vi "Set Security Level CORE.vi"(8 "error in (no error)":errorcluster, 9 "Set or Clear":T1, 10 "New Level":T2, 11 "Security System in":refnum<class "Security System.lvclass">) -> (0 "error out":errorcluster, 2 "Last Action Performed":string, 3 "Security System out":refnum<class "Security System.lvclass">)   [LabVIEW 2014, in "Security System.lvclass"]
uses:
  Security System.lvclass
  Security Level.ctl
  Set or Clear.ctl
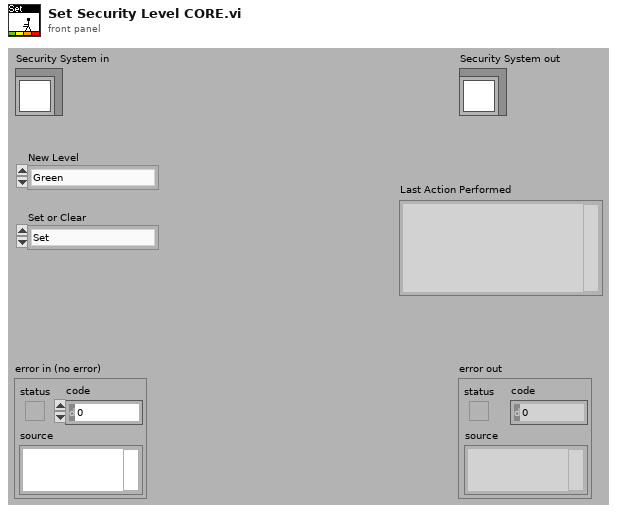
[diagram p1: front panel]
types:
  T1 = typedef "Security System.lvclass/Set or Clear.ctl" = enum16{"Set", "Clear"}
  T2 = typedef "Security System.lvclass/Security Level.ctl" = enum16{"Green", "Yellow", "Orange", "Red"}
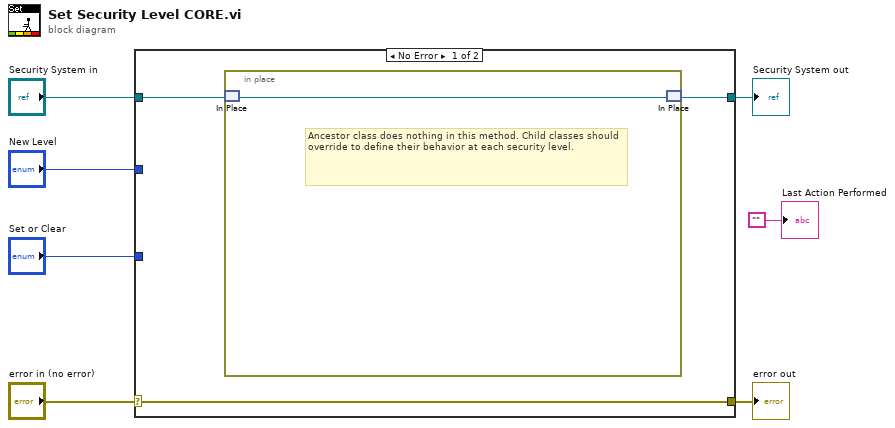
[diagram p0: block diagram]
diagram:
  n1 = case shown="No Error" "error in (no error)" {
    selector: "error in (no error)" -> [w10 w13]
    tunnel: [w10 w13] -> w6
    tunnel: [w8 w12] -> w4
    tunnel: "Security System in" -> [w9 w12]
    tunnel: "New Level" -> [_ _]
    tunnel: "Set or Clear" -> [_ _]
    frame No Error {
      n2 = in-place {
        # "Ancestor class does nothing in this method. Child classes should override to define their behavior at each security level."
        n3 = in-place-match #1(w9) -> (w11:refnum<class "Security System.lvclass">)
        n4 = in-place-match #1(w11) -> (w8:refnum<class "Security System.lvclass">)
      }
    }
    frame Error {
    }
  }
  "error out" <- w6
  "Security System out" <- w4
  "Last Action Performed" <- ""
